vi "FRCts20_Backend_GetOpenTeams.vi"(8 "error in (no error)":errorcluster, 9 "Key":string, 11 "TeamData":T2) -> (0 "error out":errorcluster)   [LabVIEW 2014, in "FRCts20_Backend_Engine_Deprecated.lvlib"]
uses:
  FRCts20_Backend_Engine_Deprecated.lvlib
  FRCts20_Backend_Engine.lvlib
  FRCts20_Backend_FGVOperation.ctl
  FRCts20_Backend_IssueDfn.ctl
  FRCts20_Backend_Controls.lvlib
  FRCts20_Backend_TeamDfn.ctl
  FRCts20_Backend_TeamDataDfn.ctl
  FRCts20_Backend_TeamList.ctl
  FRCts20_Backend_Team_Info.ctl
  FRCts20_Backend_Note.ctl
  FRCts20_Backend_Note_list.ctl
  FRCts20_Backend_request_info.ctl
  FRCts20_Backend_IssueTeamList.ctl
panel:
  in  "TeamList":T1
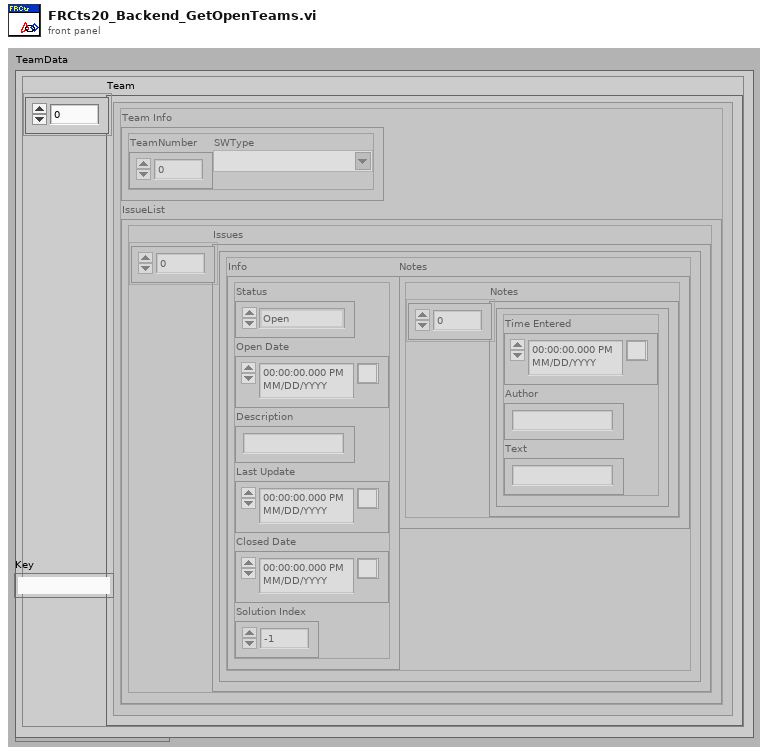
[diagram p1: front panel]
types:
  T1 = typedef "FRCts20_Backend_Controls.lvlib/FRCts20_Backend_TeamList.ctl" = cluster{"Team":cluster{"TeamNumber":u16, "Location":string}[]}
  T2 = typedef "FRCts20_Backend_Controls.lvlib/FRCts20_Backend_TeamDataDfn.ctl" = cluster{"Team":T3[]}
  T3 = typedef "FRCts20_Backend_Controls.lvlib/FRCts20_Backend_TeamDfn.ctl" = cluster{"Team Info":T4, "IssueList":T5}
  T4 = typedef "FRCts20_Backend_Controls.lvlib/FRCts20_Backend_Team_Info.ctl" = cluster{"TeamNumber":u16, "SWType":string}
  T5 = typedef "FRCts20_Backend_Controls.lvlib/FRCts20_Backend_IssueTeamList.ctl" = cluster{"Issues":T6[]}
  T6 = typedef "FRCts20_Backend_Controls.lvlib/FRCts20_Backend_IssueDfn.ctl" = cluster{"Notes":T7, "Info":T9}
  T7 = typedef "FRCts20_Backend_Controls.lvlib/FRCts20_Backend_Note_list.ctl" = cluster{"Notes":T8[]}
  T8 = typedef "FRCts20_Backend_Controls.lvlib/FRCts20_Backend_Note.ctl" = cluster{"Time Entered":timestamp, "Author":string, "Text":string}
  T9 = typedef "FRCts20_Backend_Controls.lvlib/FRCts20_Backend_request_info.ctl" = cluster{"Status":enum16{"Open", "In Work", "Closed"}, "Open Date":timestamp, "Description":string, "Last Update":timestamp, "Closed Date":timestamp, "Solution Index":i32}
  T10 = typedef "FRCts20_Backend_Engine.lvlib/FRCts20_Backend_FGVOperation.ctl" = enum16{"Initialize", "EnqueueMessage", "EnqueueDataReturn", "FlushMessage", "FlushDataReturn"}
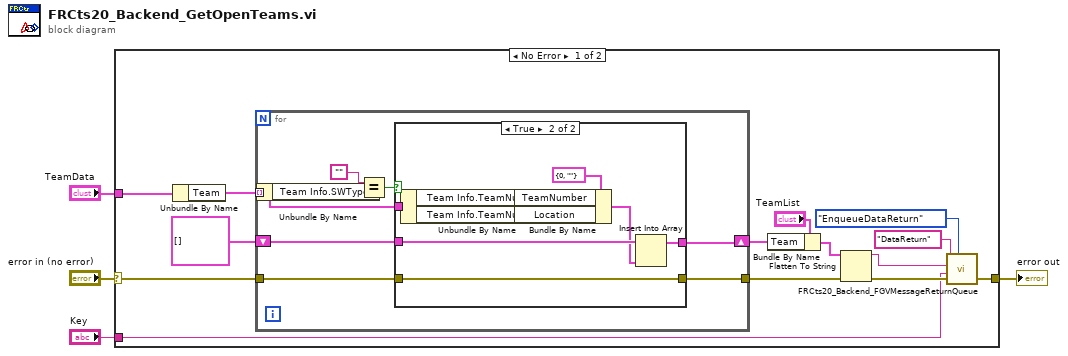
[diagram p0: block diagram]
diagram:
  n1 = case shown="No Error" "error in (no error)" {
    selector: "error in (no error)" -> [w16 w37]
    tunnel: [w9 w37] -> w3
    tunnel: "TeamData" -> [w17 _]
    tunnel: "Key" -> [w8 _]
    frame No Error {
      n2 = Unbundle By Name(w17) -> ("Team"=w18:T3[])
      n3 = for {
        tunnel: w18 -> [w23] mode=indexing
        tunnel: w16 -> [w22]
        tunnel: [w21] -> w14
        shift-right: [w19] -> w5
        shift-left: cluster{"TeamNumber":u16, "Location":string}[] [] ("Team") -> [w20]
        n4 = Unbundle By Name(w23) -> ("Team Info.SWType"=w26:string)
        n5 = Equal?(x="", y=w26) -> (x = y?=w24:bool)
        n6 = case shown="True" w24 {
          tunnel: w23 -> [_ w35]
          tunnel: w22 -> [w28 w36]
          tunnel: [w28 w36] -> w21
          tunnel: w20 -> [w27 w34]
          tunnel: [w27 w33] -> w19
          frame False {
          }
          frame True {
            n7 = Unbundle By Name(w35) -> ("Team Info.TeamNumber"=w31:u16, "Team Info.TeamNumber"=w30:u16)
            n8 = Bundle By Name(cluster=cluster{"TeamNumber":u16, "Location":string} {"TeamNumber"=0, "Location"=""} ("Team"), "TeamNumber"=w31, "Location"=w30) -> (w29:cluster{"TeamNumber":u16, "Location":string})
            n9 = Insert Into Array(array=w34, new element=w29) -> (w33:cluster{"TeamNumber":u16, "Location":string}[])  [unwired: 1 in]
          }
        }
      }
      n10 = Bundle By Name(cluster="TeamList", "Team"=w5) -> (w15:T1)
      n11 = Flatten To String(anything=w15, error in (no error)=w14) -> (data string=w10:string, error out=w11:errorcluster)  [unwired: 2 in, 1 out]
      n12 = call "FRCts20_Backend_FGVMessageReturnQueue.vi"("Operation"=FRCts20_Backend_FGVOperation."EnqueueDataReturn", "error in (no error)"=w11, "Key"=w8, "Message Value"=w10, "Message Name"="DataReturn") -> ("error out"=w9:errorcluster)  [unwired: 3 in, 1 out]
    }
    frame Error {
    }
  }
  "error out" <- w3
